vi "_DC Attenuation Tree.vi"   [LabVIEW 2011]
uses:
  LIB/DC Attenuation Version.vi
panel:
  # "See Diagram"
types:
  T1 = typedef "OGAB Version.ctl" = cluster{"Version":string, "Build Number":u32, "Build Date/Time":dbl}
  T2 = typedef "Field Record.ctl" = cluster{"ixField":i32, "iSequenceOrder":i32, "sxFieldId":string, "sxSequenceId":string, "sDisplayName":string, "sValue":string, "sUnits":string, "nDataType":T3, "nNextItem":T4, "fSystem":bool, "fSystemValue":bool, "fRequired":bool, "fSetAtTest":bool, "fTestField":bool, "fDeleted":bool, "fIndexed":bool, "fFreeList":bool}
  T3 = typedef "Field DataTypes.ctl" = enum32{"text", "numeric", "list", "timestamp", "boolean"}
  T4 = typedef "Field NextItem.ctl" = enum32{"Reset", "Retain", "Auto-Increment"}
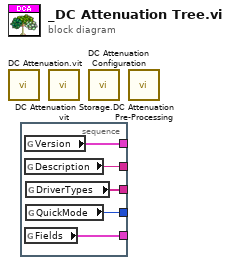
[diagram p0: block diagram]
diagram:
  n1 = call "DC Attenuation.vit"() -> ()  [unwired: 4 in, 8 out]
  n2 = stacked-sequence {
    tunnel: [w5] -> _
    tunnel: [w4] -> _
    tunnel: [w3] -> _
    tunnel: [w2] -> _
    tunnel: [w1] -> _
    frame #0 {
      n3 = global read "DC Attenuation Version.vi" "Version"() -> (w5:T1)
      n4 = global read "DC Attenuation Version.vi" "Description"() -> (w4:string)
      n5 = global read "DC Attenuation Version.vi" "Fields"() -> (w1:T2[])
      n6 = global read "DC Attenuation Version.vi" "DriverTypes"() -> (w3:string[])
      n7 = global read "DC Attenuation Version.vi" "QuickMode"() -> (w2:i32)
    }
  }
  n8 = call "DC Attenuation Storage.vit"() -> ()  [unwired: 4 in, 8 out]
  n9 = call "DC Attenuation Configuration.vi"() -> ()  [unwired: 5 in, 7 out]
  n10 = call "DC Attenuation Pre-Processing.vi"() -> ()  [unwired: 5 in, 7 out]
